vi "NewClimb.vi"   [LabVIEW 2012]
uses:
  State_Machine_Enum.ctl
  <vilib>/Rock Robotics/WPI/Solenoid/WPI_SolenoidValue.ctl
  RefnameEnum.ctl
  Robot Global Data.vi
  <vilib>/Rock Robotics/WPI/Solenoid/WPI_SolenoidSetEnum.vi
types:
  T1 = typedef "State_Machine_Enum.ctl" = enum16{"Idle", "Start", "Do", "Stop", "Init"}
  T2 = typedef "WPI_SolenoidValue.ctl" = enum16{"Off", "On", "Forward", "Reverse"}
  T3 = typedef "RefnameEnum.ctl" = enum16{"FireLauncher", "Climber", "Shield", "TankDrive", "DriveEncoderL", "DriveEncoderR", "LauncherMotorRPM", "LauncherEncoderAnalog", "LauncherEncoderRPM", "ShooterLS", "DriveAlignLS", "ClimbingLS", "LauncherEncoderAngle", "LauncherMotorAngle", "Gamepad1", "Gamepad2", "Compressor"}
  T4 = typedef "WPI_SolenoidDevRef.ctl" = cluster{"DevStatus":errorcluster, "Solenoid Module":T5, "Forward Solenoid Channel":T6, "Reverse Solenoid Channel":T6}
  T5 = typedef "FPGA_TypedefSolenoidModule.ctl" = enum16{"Solenoid Module 1", "Solenoid Module 2"}
  T6 = typedef "WPI_SolenoidChannel.ctl" = enum8{"Solenoid 1", "Solenoid 2", "Solenoid 3", "Solenoid 4", "Solenoid 5", "Solenoid 6", "Solenoid 7", "Solenoid 8", "Invalid"}
  T7 = typedef "WPI_DigitalInputDevRef.ctl" = cluster{"DevStatus":errorcluster, "DIO Channel":T8, "Digital Module":T9}
  T8 = typedef "FPGA_DIOChannel.ctl" = enum8{"DIO 1", "DIO 2", "DIO 3", "DIO 4", "DIO 5", "DIO 6", "DIO 7", "DIO 8", "DIO 9", "DIO 10", "DIO 11", "DIO 12", "DIO 13", "DIO 14", "Invalid"}
  T9 = typedef "FPGA_TypedefDigitalModule.ctl" = enum16{"Digital Module 1", "Digital Module 2"}
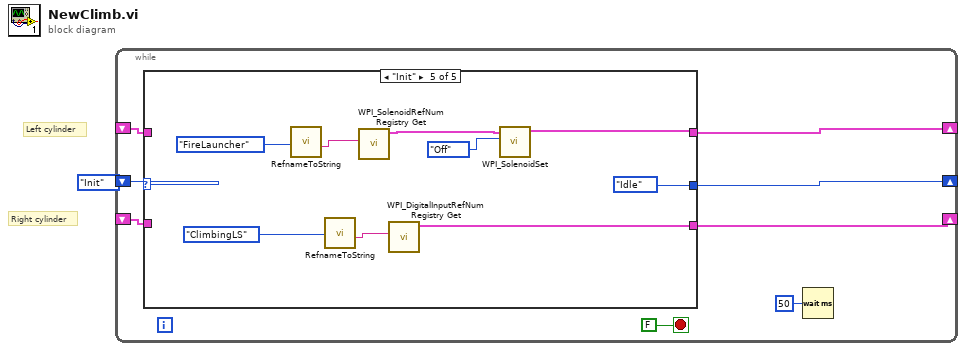
[diagram p0: block diagram]
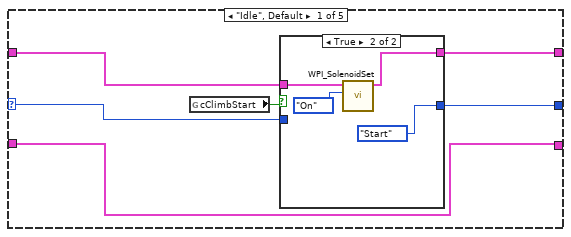
[diagram p2: hidden frame]
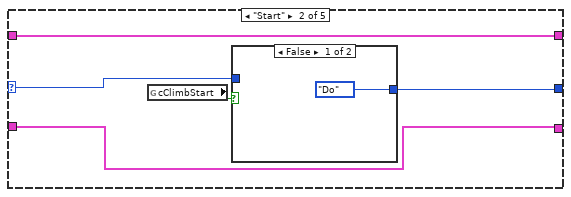
[diagram p4: hidden frame]
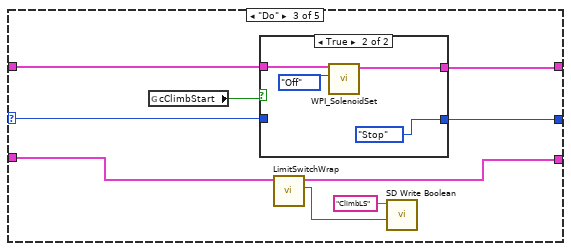
[diagram p6: hidden frame]
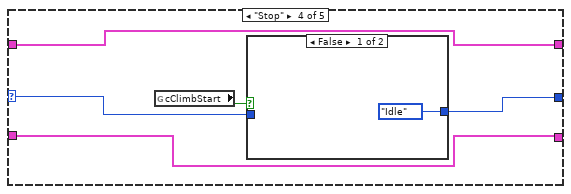
[diagram p8: hidden frame]
diagram:
  # "Right cylinder"
  # "Left cylinder"
  n1 = while {
    shift-right: [w8] -> _
    shift-left: State_Machine_Enum."Init" ("State") -> [w9]
    shift-right: [w7] -> _
    shift-left: _ -> [w6]
    shift-right: [w3] -> _
    shift-left: _ -> [w2]
    stop <- FALSE stop-if-true
    n2 = case shown="\"Init\"" w9 {
      selector: w9 -> [w11 w23 w33 w46 _]
      tunnel: [w12 w24 w34 w47 State_Machine_Enum."Idle" ("State")] -> w8
      tunnel: [w13 w26 w35 w45 w57] -> w7
      tunnel: w6 -> [w14 w26 w36 w45 _]
      tunnel: [w10 w22 w30 w44 w55] -> w3
      tunnel: w2 -> [w10 w22 w29 w44 _]
      frame "Idle", Default {
        n3 = global read "Robot Global Data.vi" "cClimbStart"() -> (w15:bool)
        n4 = case shown="True" w15 {
          tunnel: w14 -> [w16 w21]
          tunnel: [w16 w20] -> w13
          tunnel: [w17 State_Machine_Enum."Start" ("State")] -> w12
          tunnel: w11 -> [w17 _]
          frame False {
          }
          frame True {
            n5 = call-poly <vilib>:"WPI_SolenoidSet.vi"("Value"=WPI_SolenoidValue."On", "SolenoidDevRef"=w21) -> ("SolenoidDevRef"=w20:T4)  [unwired: 8 in, 1 out]
          }
        }
      }
      frame "Start" {
        n6 = global read "Robot Global Data.vi" "cClimbStart"() -> (w25:bool)
        n7 = case shown="False" w25 {
          tunnel: [State_Machine_Enum."Do" ("State") w28] -> w24
          tunnel: w23 -> [_ w28]
          frame False {
          }
          frame True {
          }
        }
      }
      frame "Do" {
        n8 = global read "Robot Global Data.vi" "cClimbStart"() -> (w37:bool)
        n9 = case shown="True" w37 {
          tunnel: w36 -> [w39 w43]
          tunnel: [w39 w42] -> w35
          tunnel: [w38 State_Machine_Enum."Stop" ("State")] -> w34
          tunnel: w33 -> [w38 _]
          frame False {
          }
          frame True {
            n10 = call-poly <vilib>:"WPI_SolenoidSet.vi"("Value"=WPI_SolenoidValue."Off", "SolenoidDevRef"=w43) -> ("SolenoidDevRef"=w42:T4)  [unwired: 8 in, 1 out]
          }
        }
        n11 = call "LimitSwitchWrap.vi"("DigitalInputDevRef"=w29) -> ("Triggered"=w32:bool, "DigitalInputDevRef 2"=w30:T7)  [unwired: 9 in]
        n12 = call <vilib>:"SD Write Boolean.vi"("Boolean"=w32, "Name"="ClimbLS") -> ()  [unwired: 8 in, 2 out]
      }
      frame "Stop" {
        n13 = global read "Robot Global Data.vi" "cClimbStart"() -> (w48:bool)
        n14 = case shown="False" w48 {
          tunnel: [State_Machine_Enum."Idle" ("State") w50] -> w47
          tunnel: w46 -> [_ w50]
          frame False {
          }
          frame True {
          }
        }
      }
      frame "Init" {
        n15 = call "RefnameToString.vi"("Enum"=RefnameEnum."FireLauncher") -> ("Refname"=w53:string)  [unwired: 10 in]
        n16 = call "RefnameToString.vi"("Enum"=RefnameEnum."ClimbingLS") -> ("Refname"=w51:string)  [unwired: 10 in]
        n17 = call <vilib>:"WPI_SolenoidRefNum Registry Get.vi"("refnum name"=w53) -> ("SolenoidDevRef"=w58:T4)  [unwired: 9 in, 1 out]
        n18 = call <vilib>:"WPI_DigitalInputRefNum Registry Get.vi"("refnum name"=w51) -> ("DigitalInputDevRef"=w55:T7)  [unwired: 9 in, 1 out]
        n19 = call-poly <vilib>:"WPI_SolenoidSet.vi"("Value"=WPI_SolenoidValue."Off", "SolenoidDevRef"=w58) -> ("SolenoidDevRef"=w57:T4)  [unwired: 8 in, 1 out]
      }
    }
    n20 = Wait (ms)(milliseconds to wait=u32 50) -> ()  [unwired: 1 out]
  }
